vi "Calc_Sum_of_Samples_DBL.vi"(1 "Reset?":bool, 2 "Input sample":dbl format="%#_13g") -> (0 "Sum of samples":dbl)   [LabVIEW 2018, in "TTL IO.lvlib"]
uses:
  TTL IO.lvlib
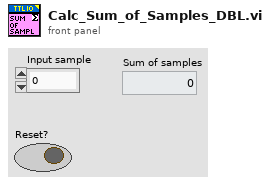
[diagram p1: front panel]
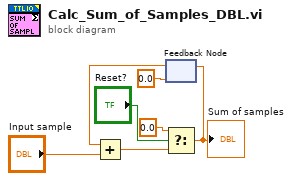
[diagram p0: block diagram]
diagram:
  n1 = feedback #1(0.0) -> (w2:dbl)
  n2 = Add(x=w2, y="Input sample") -> (x+y=w4:dbl)
  n3 = Select(t=0.0, s="Reset?", f=w4) -> (s? t:f=w3:dbl)
  "Sum of samples" <- w3
  n4 = feedback-in #1(w3) -> ()
